vi "Volume_Control.vi"(9 "z (m)":dbl, 10 "y (m)":dbl, 11 "x (m)":dbl) -> (2 "Range acceptable?":bool)   [LabVIEW 2015]
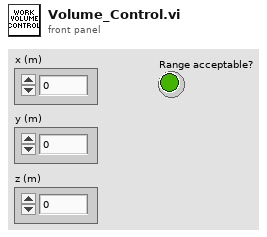
[diagram p1: front panel]
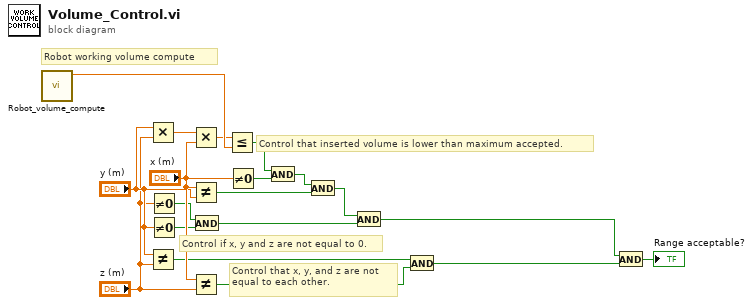
[diagram p0: block diagram]
diagram:
  # "Control that inserted volume is lower than maximum accepted."
  # "Control that x, y, and z are not equal to each other."
  # "Control if x, y and z are not equal to 0."
  # "Robot working volume compute"
  n1 = call "Robot_volume_compute.vi"() -> ("Volume (m^3)"=w19:dbl)  [unwired: 11 in]
  n2 = Multiply(x="y (m)", y="z (m)") -> (x*y=w18:dbl)
  n3 = Not Equal?(x="y (m)", y="z (m)") -> (x != y?=w3:bool)
  n4 = Not Equal To 0?(x="z (m)") -> (x != 0?=w9:bool)
  n5 = Not Equal To 0?(x="y (m)") -> (x != 0?=w8:bool)
  n6 = Multiply(x=w18, y="x (m)") -> (x*y=w17:dbl)
  n7 = Not Equal?(x="x (m)", y="y (m)") -> (x != y?=w10:bool)
  n8 = Not Equal?(x="x (m)", y="z (m)") -> (x != y?=w2:bool)
  n9 = And(x=w9, y=w8) -> (x .and. y?=w6:bool)
  n10 = Less Or Equal?(x=w17, y=w19) -> (x <= y?=w16:bool)
  n11 = Not Equal To 0?(x="x (m)") -> (x != 0?=w15:bool)
  n12 = And(x=w16, y=w15) -> (x .and. y?=w14:bool)
  n13 = And(x=w14, y=w10) -> (x .and. y?=w7:bool)
  n14 = And(x=w7, y=w6) -> (x .and. y?=w5:bool)
  n15 = And(x=w3, y=w2) -> (x .and. y?=w1:bool)
  n16 = And(x=w5, y=w1) -> (x .and. y?=→"Range acceptable?":bool)
